vi "Set VI Breakpoints.vi"(8 "error in":errorcluster, 9 "Breakpoints":T2[](array[typedef]), 10 "Class Name":T1=enum."Wire", 11 "VI Reference in":refnum<vi>) -> (0 "error out":errorcluster, 2 "VI Modified":bool, 3 "VI Reference out":refnum<vi>)   [LabVIEW 2020]
doc: "This VI sets breakpoint statuses for the specified class in the active VI."
uses:
  Type Definitions/Breakpoint--cluster.ctl
  <vilib>/Utility/miscctls.llb/LVBreakpointStatusEnum.ctl
  Type Definitions/Class Name--enum.ctl
  <vilib>/Utility/traverseref.llb/TRef TravTarget.ctl
  <vilib>/Utility/traverseref.llb/VI Scripting - Traverse.lvlib
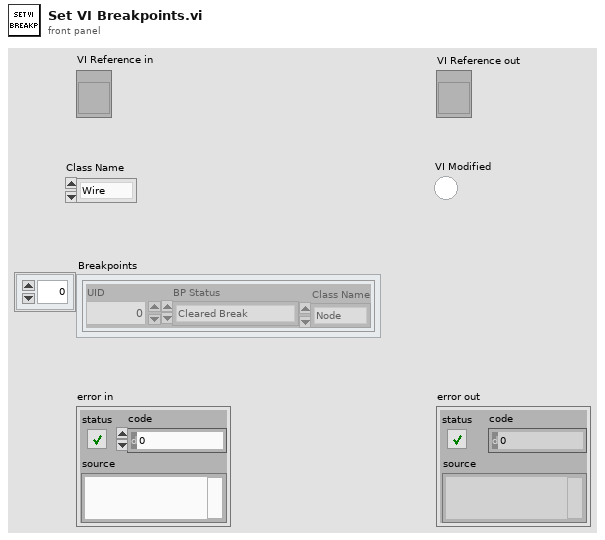
[diagram p1: front panel]
types:
  T1 = typedef "Class Name--enum.ctl" = enum16{"Node", "Wire"}
  T2 = typedef "Breakpoint--cluster.ctl" = cluster{"UID":i32, "BP Status":T3, "Class Name":T1}
  T3 = typedef "LVBreakpointStatusEnum.ctl" = enum8{"Cleared Break", "Enabled Break", "Disabled Break"}
  T4 = typedef "TRef TravTarget.ctl" = enum16{"FP", "BD", "Other"}
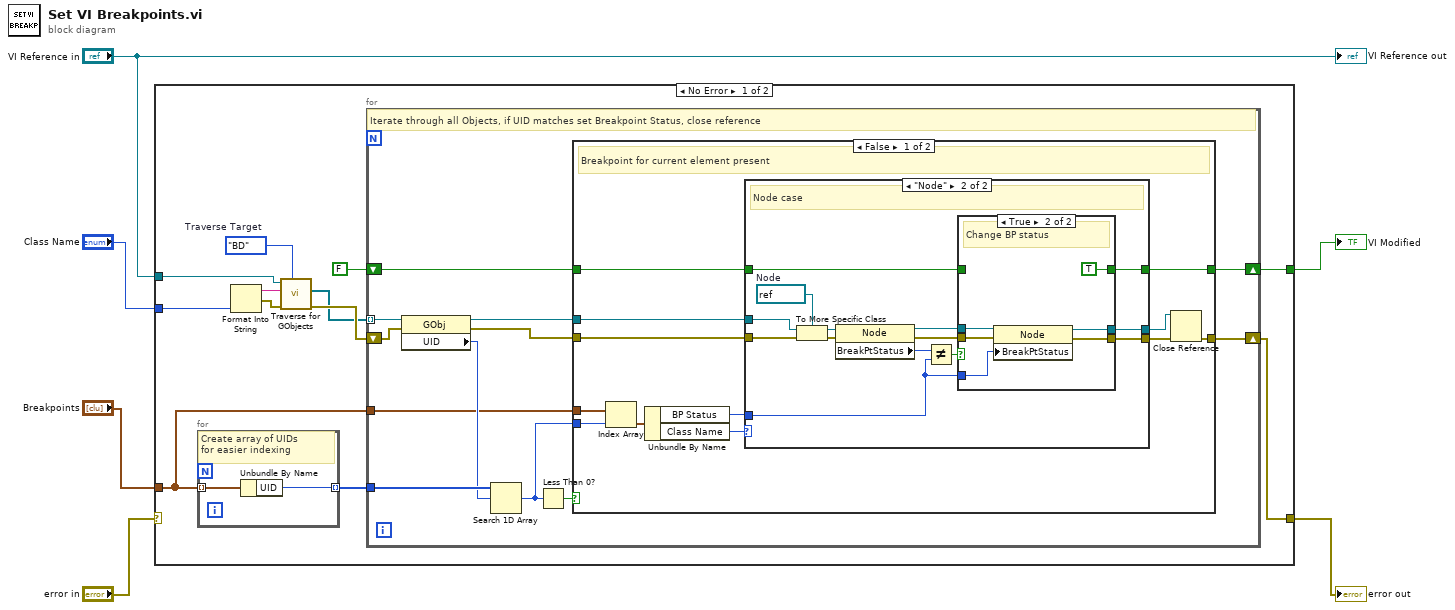
[diagram p0: block diagram]
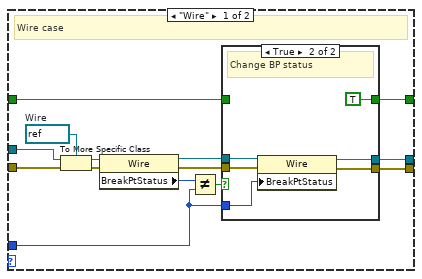
[diagram p2: hidden frame]
diagram:
  n1 = case shown="No Error" "error in" {
    selector: "error in" -> [_ w93]
    tunnel: "VI Reference in" -> [w11 _]
    tunnel: [w18 w93] -> w5
    tunnel: "Breakpoints" -> [w14 _]
    tunnel: "Class Name" -> [w9 _]
    tunnel: [w7 _] -> w1
    frame No Error {
      w13 = TRef_TravTarget."BD"  # Traverse Target
      n2 = for {
        tunnel: w14 -> [w20] mode=indexing
        tunnel: [w19] -> w15 mode=indexing
        # "Create array of UIDs\nfor easier indexing"
        n3 = Unbundle By Name(w20) -> ("UID"=w19:i32)
      }
      n4 = Format Into String(w9) -> (resulting string=w12:string, error out=w17:errorcluster)  [unwired: 3 in]
      n5 = call <vilib>:"Traverse for GObjects.vi"("Traverse Target"=w13, "error in (no error)"=w17, "Class Name"=w12, "VI Refnum"=w11) -> ("error out"=w16:errorcluster, "References"=w10:refnum<vi>[])  [unwired: 4 in, 2 out]
      n6 = for {
        shift-right: [w32] -> w18
        shift-left: w16 -> [w31]
        tunnel: w10 -> [w29] mode=indexing
        tunnel: w15 -> [w28]
        tunnel: w14 -> [w25]
        shift-right: [w21] -> w7
        shift-left: FALSE -> [w22]
        # "Iterate through all Objects, if UID matches set Breakpoint Status, close reference"
        n7 = property class="GObj"(reference=w29, error in=w31) -> (reference out=w23:refnum<vi>, error out=w30:errorcluster, "UID"=w27:i32)
        n8 = Search 1D Array(1D array=w28, element=w27) -> (index of element=w24:i32)  [unwired: 1 in]
        n9 = Less Than 0?(x=w24) -> (x < 0?=w26:bool)
        n10 = case shown="False" w26 {
          tunnel: [w43 w92] -> w32
          tunnel: w25 -> [w40 _]
          tunnel: w24 -> [w39 _]
          tunnel: w23 -> [w38 _]
          tunnel: w30 -> [w42 w92]
          tunnel: w22 -> [w33 w91]
          tunnel: [w34 w91] -> w21
          frame False {
            # "Breakpoint for current element present"
            n11 = Index Array(array=w40, index=w39) -> (element=w37:T2)
            n12 = Unbundle By Name(w37) -> ("BP Status"=w35:T3, "Class Name"=w36:T1)
            n13 = case shown="\"Node\"" w36 {
              tunnel: w38 -> [w54 w77]
              tunnel: w42 -> [w58 w81]
              tunnel: [w56 w79] -> w44
              tunnel: [w53 w76] -> w41
              tunnel: w35 -> [w47 w71]
              tunnel: [w46 w70] -> w34
              tunnel: w33 -> [w45 w69]
              frame "Wire" {
                w52 = refnum<vi> refnum  # Wire
                # "Wire case"
                n14 = To More Specific Class(target class=w52, reference=w54, error in=w58) -> (specific class reference=w51:refnum<vi>, error out=w57:errorcluster)
                n15 = property class="Wire"(reference=w51, error in=w57) -> (reference out=w50:refnum<vi>, error out=w55:errorcluster, "BreakPtStatus"=w49:T3)
                n16 = Not Equal?(x=w49, y=w47) -> (x != y?=w48:bool)
                n17 = case shown="True" w48 {
                  tunnel: [w61 w67] -> w56
                  tunnel: [w60 w65] -> w53
                  tunnel: w55 -> [w61 w66]
                  tunnel: w50 -> [w60 w64]
                  tunnel: w47 -> [_ w63]
                  tunnel: [w59 TRUE] -> w46
                  tunnel: w45 -> [w59 _]
                  frame False {
                    # "No change needed"
                  }
                  frame True {
                    # "Change BP status"
                    n18 = property class="Wire"(reference=w64, error in=w66, "BreakPtStatus"=w63) -> (reference out=w65:refnum<vi>, error out=w67:errorcluster)
                  }
                }
              }
              frame "Node" {
                w68 = refnum<vi> refnum  # Node
                # "Node case"
                n19 = To More Specific Class(target class=w68, reference=w77, error in=w81) -> (specific class reference=w75:refnum<vi>, error out=w80:errorcluster)
                n20 = property class="Node"(reference=w75, error in=w80) -> (reference out=w74:refnum<vi>, error out=w78:errorcluster, "BreakPtStatus"=w73:T3)
                n21 = Not Equal?(x=w73, y=w71) -> (x != y?=w72:bool)
                n22 = case shown="True" w72 {
                  tunnel: [w84 w90] -> w79
                  tunnel: [w83 w88] -> w76
                  tunnel: w78 -> [w84 w89]
                  tunnel: w74 -> [w83 w87]
                  tunnel: w71 -> [_ w86]
                  tunnel: [w82 TRUE] -> w70
                  tunnel: w69 -> [w82 _]
                  frame False {
                    # "No change needed"
                  }
                  frame True {
                    # "Change BP status"
                    n23 = property class="Node"(reference=w87, error in=w89, "BreakPtStatus"=w86) -> (reference out=w88:refnum<vi>, error out=w90:errorcluster)
                  }
                }
              }
            }
            n24 = Close Reference(reference=w41, error in (no error)=w44) -> (error out=w43:errorcluster)
          }
          frame True {
            # "No breakpoint for present element"
          }
        }
      }
    }
    frame Error {
      # "Pass error without further action"
    }
  }
  "error out" <- w5
  "VI Modified" <- w1
  "VI Reference out" <- "VI Reference in"
